vi "Global 1.vi"() -> ()   [LabVIEW 2015]
panel:
  in  "Cluster":cluster{"bol1":bool, "Num1":dbl}
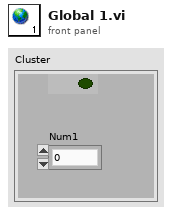
[diagram p1: front panel]
diagram:
